vi "Test Info.vi"(8 "error in (no error)":errorcluster, 10 "Test info":T1, 11 "Access in":refnum<class "Access.lvclass">) -> (0 "error out":errorcluster, 3 "Access out":refnum<class "Access.lvclass">)   [LabVIEW 2021, in "Database.lvlib" / "Access.lvclass"]
uses:
  Access.lvclass
  User Interface/Test Info.ctl
  Access.lvclass/Access.ctl
  <vilib>/addons/database/NI_Database_API.lvlib
  User Interface/User Interface.lvlib
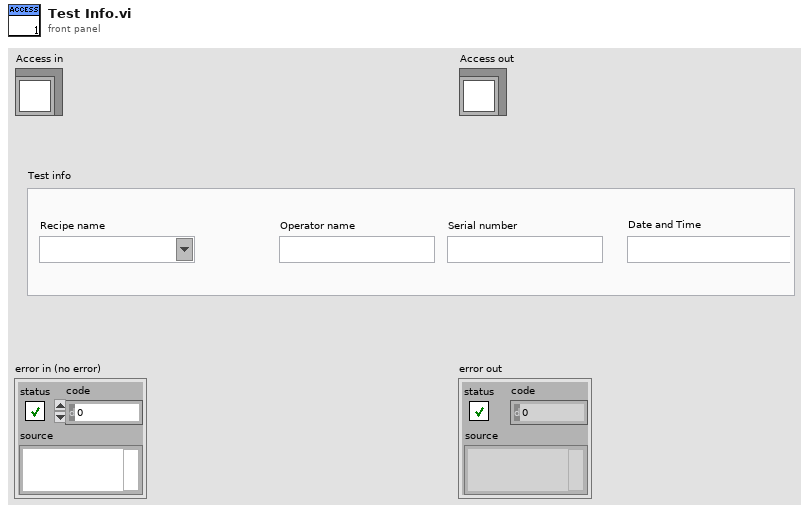
[diagram p1: front panel]
types:
  T1 = typedef "User Interface.lvlib/Test Info.ctl" = cluster{"Date and Time":string, "Recipe name":string, "Serial number":string, "Operator name":string}
  T2 = typedef "Database.lvlib/DB.lvclass/Table_info.ctl" = cluster{"Authentication":string, "Instr_Configuration":string, "Recipe":string, "Test_data":string}
  T3 = typedef "NI_Database_API.lvlib/Conn ObjectReference.ctl" = refnum<k1>
  T4 = cluster{"[0]":string, "[1]":string, "[2]":string, "[3]":string, "[4]":string, "[5]":string, "[6]":string, "[7]":string, "[8]":string, "[9]":string, "[10]":string, "[11]":string, "[12]":string, "[13]":string}
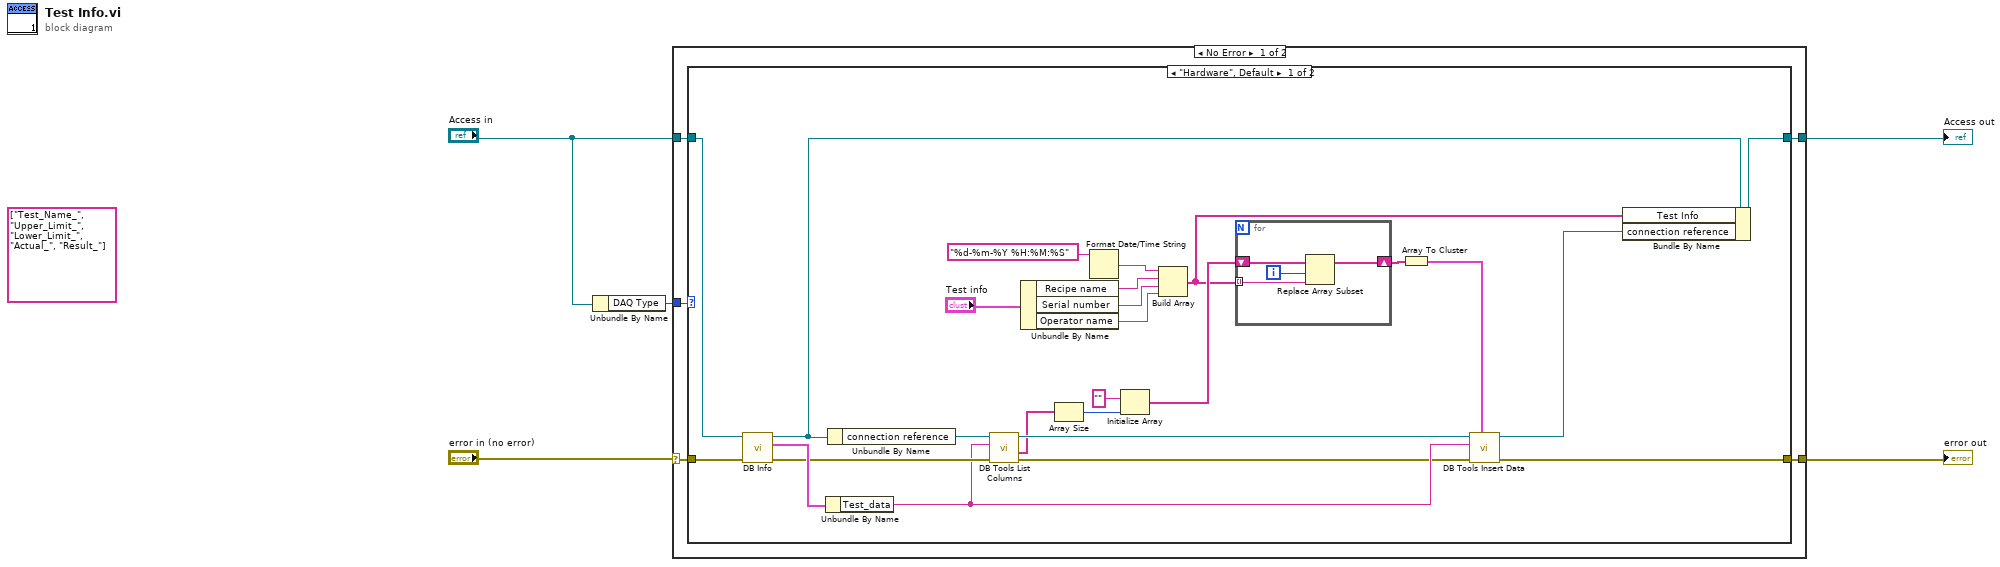
[diagram p0: block diagram]
diagram:
  (unwired) string[] ["Test_Name_", "Upper_Limit_", "Lower_Limit_", "Actual_", "Result_"]
  n1 = Unbundle By Name("Access in") -> ("DAQ Type"=w5:enum16{"Hardware", "Simulation"})
  n2 = case shown="No Error" "error in (no error)" {
    selector: "error in (no error)" -> [w7 w42]
    tunnel: "Access in" -> [w9 w43]
    tunnel: w5 -> [w10 _]
    tunnel: [w8 w43] -> w1
    tunnel: [w6 w42] -> w2
    frame No Error {
      n3 = case shown="\"Hardware\", Default" w10 {
        tunnel: w9 -> [w34 w41]
        tunnel: [w31 w41] -> w8
        tunnel: w7 -> [w33 w40]
        tunnel: [w29 w40] -> w6
        frame "Hardware", Default {
          n4 = call-dynamic "DB Info.vi"("error in (no error)"=w33, "Access in"=w34) -> ("error out"=w28:errorcluster, "Table_info"=w32:T2, "Access out"=w27:refnum<class "Access.lvclass">)  [unwired: 6 in, 1 out]
          n5 = Unbundle By Name(w32) -> ("Test_data"=w25:string)
          n6 = Unbundle By Name(w27) -> ("connection reference"=w26:T3)
          n7 = call <vilib>:"DB Tools List Columns.vi"("error in (no error)"=w28, "table"=w25, "connection reference"=w26) -> ("error out"=w24:errorcluster, "columns"=w22:string[], "connection reference out"=w23:T3)  [unwired: 1 in, 1 out]
          n8 = Unbundle By Name("Test info") -> ("Recipe name"=w18:string, "Serial number"=w17:string, "Operator name"=w16:string)
          n9 = Array Size(array=w22) -> (size(s)=w21:i32)
          n10 = Format Date/Time String(time format string (%c)="%d-%m-%Y %H:%M:%S") -> (date/time string=w19:string)  [unwired: 2 in]
          n11 = Initialize Array("", w21) -> (w14:string[])
          n12 = Build Array(w19, w18, w17, w16) -> (w12:string[])
          n13 = for {
            tunnel: w12 -> [w38] mode=indexing
            shift-right: [w37] -> w13
            shift-left: w14 -> [w36]
            i -> [w39]
            n14 = Replace Array Subset(array=w36, new element=w38, index=w39) -> (w37:string[])
          }
          n15 = Array To Cluster(array=w13) -> (cluster=w15:T4)
          n16 = call <vilib>:"DB Tools Insert Data.vi"("data"=w15, "error in (no error)"=w24, "table"=w25, "connection reference"=w23) -> ("error out"=w29:errorcluster, "connection reference out"=w30:T3)  [unwired: 6 in]
          n17 = Bundle By Name(cluster=w27, "Test Info"=w12, "connection reference"=w30) -> (w31:refnum<class "Access.lvclass">)
        }
        frame "Simulation" {
        }
      }
    }
    frame Error {
    }
  }
  "error out" <- w2
  "Access out" <- w1
